vi "Configure Correction.vi"(5 "Load Type (0: Cp-D)":u16(ring) items=["Cp-D", "Cp-Q", "Cp-G", "Cp-Rp", "Cs-D", "Cs-Q", "Cs-Rs", "Lp-D", "Lp-Q", "Lp-G", "Lp-Rp", "Ls-D", "Ls-Q", "Ls-Rs", "R-X", "Z-thd", "Z-thr", "G-B", "Y-thd", "Y-thr"], 7 "Channel Number (0)":i32, 8 "error in (no error)":errorcluster, 9 "Correction Mode (0: Single)":u16(ring) items=["Single", "Multiple"], 10 "Cable Length (0: 0 m)":u16(ring) items=["0 m"=0, "1 m"=1, "2 m"=2, "4 m"=4], 11 "VISA resource name":refnum<visa-resource-name>) -> (0 "error out":errorcluster, 3 "VISA resource name out":refnum<visa-resource-name>)   [LabVIEW 2016, in "Agilent E4980.lvlib"]
doc: "Configures cable length, correction mode, the measurement function for load correction, and the channel number."
uses:
  <instrlib>/Agilent E4980/Agilent E4980.lvlib
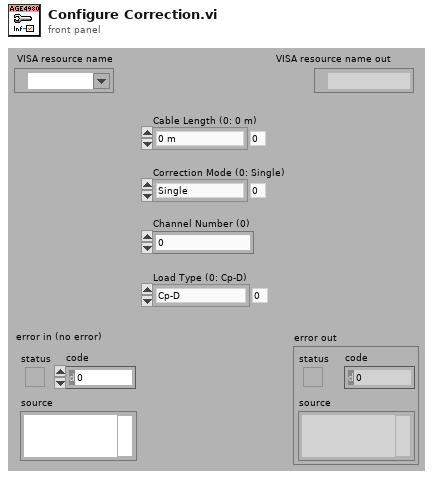
[diagram p1: front panel]
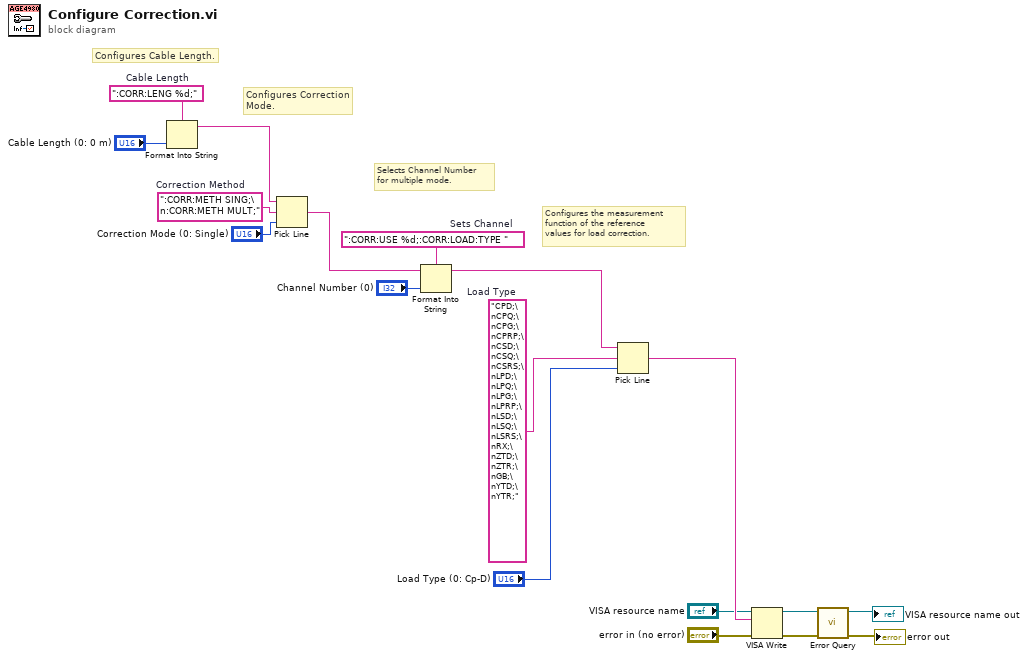
[diagram p0: block diagram]
diagram:
  w17 = "CPD;\nCPQ;\nCPG;\nCPRP;\nCSD;\nCSQ;\nCSRS;\nLPD;\nLPQ;\nLPG;\nLPRP;\nLSD;\nLSQ;\nLSRS;\nRX;\nZTD;\nZTR;\nGB;\nYTD;\nYTR;"  # Load Type
  w8 = ":CORR:USE %d;:CORR:LOAD:TYPE "  # Sets Channel
  w18 = ":CORR:METH SING;\n:CORR:METH MULT;"  # Correction Method
  w4 = ":CORR:LENG %d;"  # Cable Length
  # "Configures the measurement\nfunction of the reference\nvalues for load correction."
  # "Selects Channel Number\nfor multiple mode."
  # "Configures Correction\nMode."
  # "Configures Cable Length."
  n1 = Format Into String(format string=w4, "Cable Length (0: 0 m)") -> (resulting string=w2:string)  [unwired: 2 in, 1 out]
  n2 = Pick Line(string ("")=w2, multi-line string=w18, line index="Correction Mode (0: Single)") -> (output string=w6:string)
  n3 = Format Into String(format string=w8, initial string=w6, "Channel Number (0)") -> (resulting string=w5:string)  [unwired: 1 in, 1 out]
  n4 = Pick Line(string ("")=w5, multi-line string=w17, line index="Load Type (0: Cp-D)") -> (output string=w15:string)
  n5 = VISA Write(VISA resource name="VISA resource name", write buffer=w15, error in (no error)="error in (no error)") -> (VISA resource name out=w12:refnum<visa-resource-name>, error out=w11:errorcluster)  [unwired: 1 out]
  n6 = call <instrlib>:"Error Query.vi"("error in (no error)"=w11, "VISA resource name"=w12) -> ("error out"=→"error out":errorcluster, "VISA resource name out"=→"VISA resource name out":refnum<visa-resource-name>)  [unwired: 6 in, 2 out]
